vi "Enable Lossy.vi"(10 "Channel Data In":T1) -> (2 "Channel Data":T1)   [LabVIEW 2022 SP3, in "Flex.lvlib"]
uses:
  Flex.lvlib
  Channel Data.ctl
  Event Data.ctl
  Element.ctl
  Writer Data.ctl
  Queue Data.ctl
  Element Info.ctl
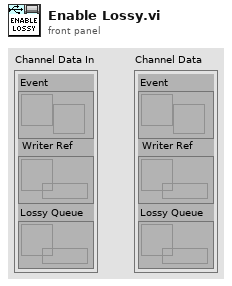
[diagram p1: front panel]
types:
  T1 = typedef "Flex.lvlib/Channel Data.ctl" = cluster{"Event":refnum<user-event>, "Writer Ref":refnum<data-value>, "Lossy Queue":refnum<queue>}
  T2 = typedef "Flex.lvlib/Writer Data.ctl" = cluster{"Lossless":refnum<queue>[], "Events":bool, "Lossy":bool}
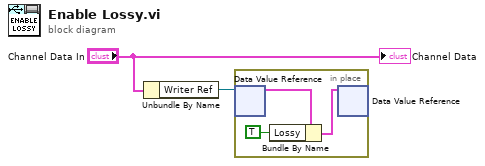
[diagram p0: block diagram]
diagram:
  n1 = Unbundle By Name("Channel Data In") -> ("Writer Ref"=w2:refnum<data-value>)
  n2 = in-place {
    n3 = in-place-dvr #1(w2) -> (w5:T2)  [unwired: 1 out]
    n4 = Bundle By Name(cluster=w5, "Lossy"=TRUE) -> (w3:T2)
    n5 = in-place-dvr #1(w3) -> ()  [unwired: 2 out]
  }
  "Channel Data" <- "Channel Data In"
